vi "extractADCSubstring.vi"(8 "error in (no error)":errorcluster, 9 "lastIsTrue?":bool, 11 "ILC in":refnum<class "ILC.lvclass">) -> (0 "error out":errorcluster, 2 "adcElement":i32, 3 "ILC out":refnum<class "ILC.lvclass">)   [LabVIEW 2013, in "ILCCommon.lvlib" / "ILC.lvclass"]
uses:
  <userlib>/Common/ILC/ILC/ILC.lvclass
  <userlib>/Common/ILC/ILCModelTypedefs/FinalDelimiter.ctl
  <userlib>/Common/ILC/ILC/ILC.lvclass/ILC.ctl
  <userlib>/Common/ILC/ILCModelTypedefs/ILCModelTypedefs.lvlib
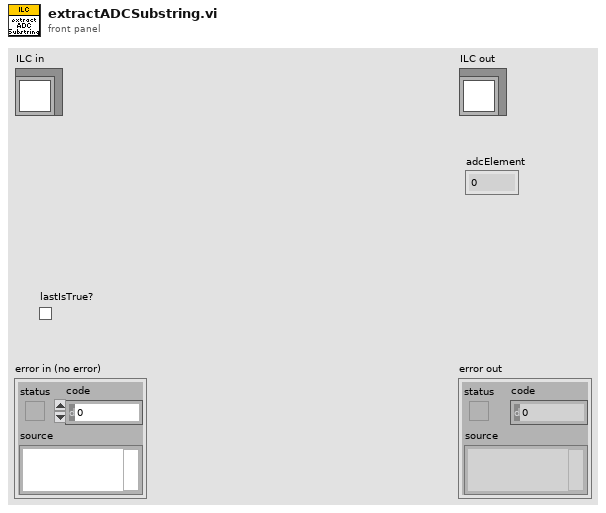
[diagram p1: front panel]
types:
  T1 = typedef "ILCCommon.lvlib/ILCModelTypedefs.lvlib/FinalDelimiter.ctl" = enum16{",", "<CR><LF>"}
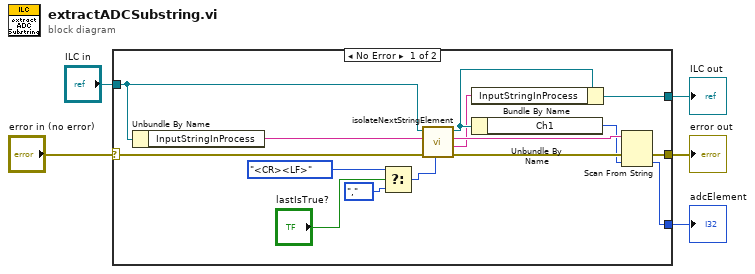
[diagram p0: block diagram]
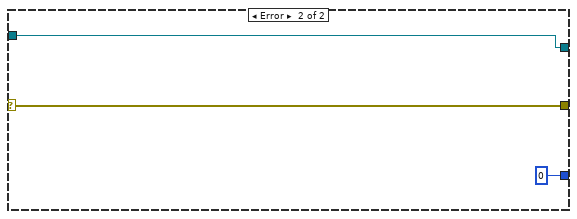
[diagram p2: hidden frame]
diagram:
  n1 = case shown="No Error" "error in (no error)" {
    selector: "error in (no error)" -> [w16 w23]
    tunnel: [w15 w23] -> w4
    tunnel: [w17 w22] -> w2
    tunnel: "ILC in" -> [w13 w22]
    tunnel: [w10 0 ("Ch1")] -> w1
    frame No Error {
      n2 = Unbundle By Name(w13) -> ("InputStringInProcess"=w14:string)
      n3 = Select(t=FinalDelimiter."<CR><LF>", s="lastIsTrue?", f=FinalDelimiter."," ("Final Delimiter")) -> (s? t:f=w6:T1)
      n4 = call <userlib>:"isolateNextStringElement.vi"("Final Delimiter"=w6, "error in (no error)"=w16, "inputString"=w14, "ILC in"=w13) -> ("error out"=w19:errorcluster, "remainingString"=w11:string, "extractedSegment"=w20:string, "ILC out"=w12:refnum<class "ILC.lvclass">)  [unwired: 4 in]
      n5 = Bundle By Name(cluster=w12, "InputStringInProcess"=w11) -> (w17:refnum<class "ILC.lvclass">)
      n6 = Unbundle By Name(w12) -> ("Ch1"=w18:i32)
      n7 = Scan From String(input string=w20, error in=w19, default 1=w18) -> (error out=w15:errorcluster, output 1=w10:i32)  [unwired: 2 in, 2 out]
    }
    frame Error {
    }
  }
  "error out" <- w4
  "ILC out" <- w2
  "adcElement" <- w1
